vi "Centauro Service Mode Display Checker.vi"(6 "Loop Rate (ms)":u32=250, 7 "Timeout (s)":dbl=5.0 format="%#_13g", 8 "Error In":errorcluster, 9 "Erd_UiLedBitmap ERD #":T1={"ERD Number"=61729, "Data Type"=enum."string"} {"ERD Number" format="%.0x"}, 10 "UI GEA Inputs":T5={"Source"=228, "Destination"=37} {"Destination" format="%.0x"; "Source" format="%.0x"}, 11 "GEA2 Reference In":refnum<k24>) -> (0 "Error Out":errorcluster, 1 "Report Text":string, 2 "LED Status Out":T4, 3 "GEA2 Reference Out":refnum<k24>)   [LabVIEW 2016]
uses:
  Common/LabVIEW GEA2 Toolkit/LabVIEW_GEA2_Toolkit.lvlibp/type defs/Source_Destination.ctl
  Q:/Common/DLLs/GEA3/GeaCommunication.dll
  Common/DLLs/GEA3/GeaCommunication.dll
  Centauro Washer/Product Testcode/Centauro/Valew Common/type defs/LED Status OOB.ctl
  Common/LabVIEW GEA2 Toolkit/LabVIEW_GEA2_Toolkit.lvlibp/type defs/ERD Read Data In.ctl
  Common/LabVIEW GEA2 Toolkit/LabVIEW_GEA2_Toolkit.lvlibp/type defs/Data Type.ctl
  Common/LabVIEW GEA2 Toolkit/LabVIEW_GEA2_Toolkit.lvlibp
panel:
  in  "Board Index":i32
  in  "LED Status Cluster":T4
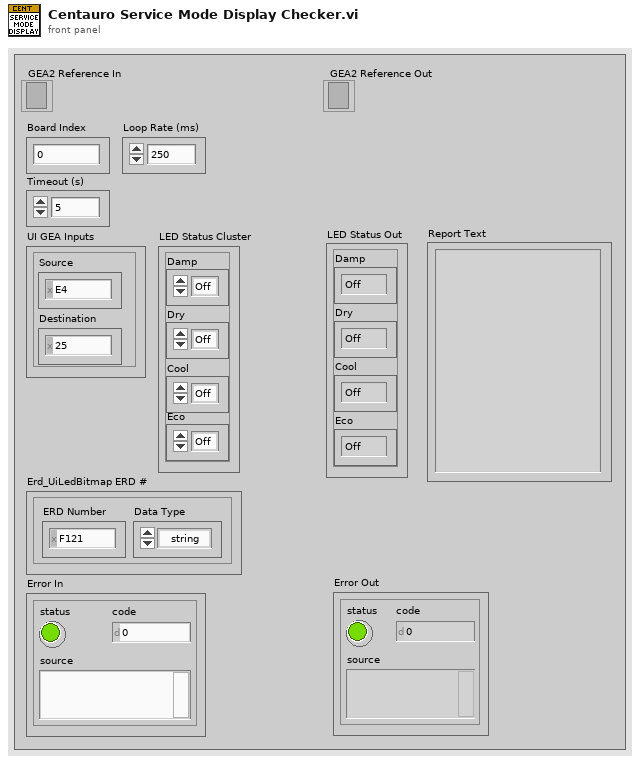
[diagram p1: front panel]
types:
  T1 = typedef "LabVIEW_GEA2_Toolkit.lvlibp/ERD Read Data In.ctl" = cluster{"ERD Number":u16, "Data Type":T2}
  T2 = typedef "LabVIEW_GEA2_Toolkit.lvlibp/Data Type.ctl" = enum16{"string", "boolean", "uint8_t", "uint16_t", "uint32_t", "uint64_t", "int8_t", "int16_t", "int32_t", "int64_t"}
  T3 = typedef "LED Status OOB.ctl" = enum32{"Off", "On", "Blink"}
  T4 = cluster{"Damp":T3, "Dry":T3, "Cool":T3, "Eco":T3}
  T5 = typedef "LabVIEW_GEA2_Toolkit.lvlibp/Source_Destination.ctl" = cluster{"Source":u8, "Destination":u8}
  T6 = enum16{"EQ (==)", "NE (!=)", "GT (>)", "LT (<)", "GE (>=)", "LE (<=)", "GTLT(> <)", "GELE (>= <=)", "GELT (>= <)", "GTLE (> <=)", "LTGT (< >)", "LEGE (<= >=)", "LEGT (<= >)", "LTGE (< >=)", "No Comparison"}
  T7 = typedef "LabVIEW_GEA2_Toolkit.lvlibp/ERD Read Data Out.ctl" = cluster{"ERD Number":u16, "Data":string}
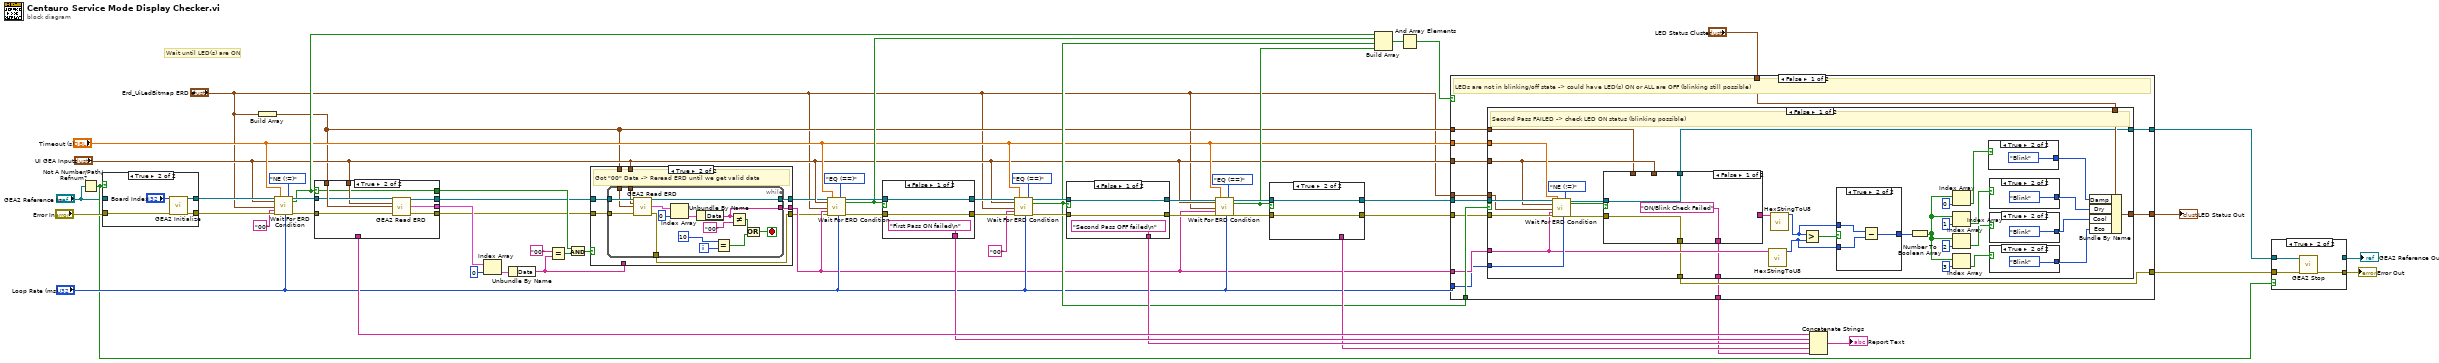
[diagram p0: block diagram]
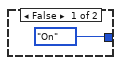
[diagram p4: hidden frame]
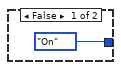
[diagram p5: hidden frame]
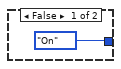
[diagram p6: hidden frame]
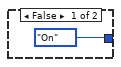
[diagram p7: hidden frame]
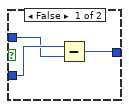
[diagram p8: hidden frame]
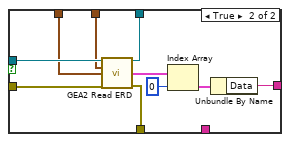
[diagram p9: hidden frame]
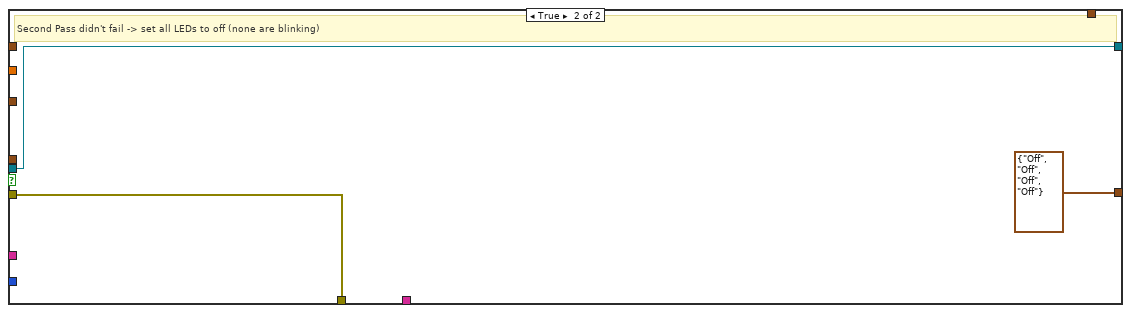
[diagram p10: hidden frame]
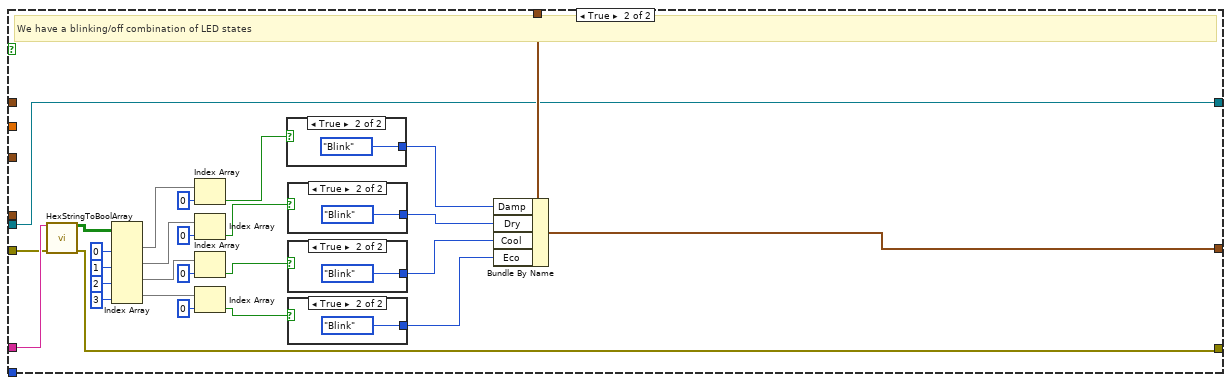
[diagram p11: hidden frame]
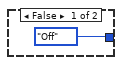
[diagram p12: hidden frame]
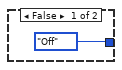
[diagram p13: hidden frame]
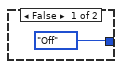
[diagram p14: hidden frame]
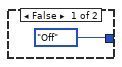
[diagram p15: hidden frame]
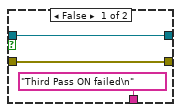
[diagram p16: hidden frame]
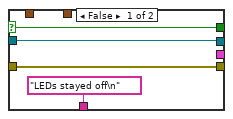
[diagram p20: hidden frame]
diagram:
  # "Wait until LED(s) are ON"
  n1 = Not A Number/Path/Refnum?(number/path/refnum="GEA2 Reference In") -> (NaN/Path/Refnum?=w2:bool)
  n2 = case shown="True" w2 {
    tunnel: [w62 w67] -> w53
    tunnel: "Error In" -> [w62 w66]
    tunnel: [w63 w65] -> w54
    tunnel: "GEA2 Reference In" -> [w63 _]
    frame False {
    }
    frame True {
      n3 = call "GEA2 Initialize.vi"("Board Index"="Board Index", "error in"=w66) -> ("GEA2 Reference Out"=w65:refnum<k24>, "error out"=w67:errorcluster)  [unwired: 11 in, 1 out]
    }
  }
  n4 = Build Array("Erd_UiLedBitmap ERD #") -> (w4:T1[])
  n5 = call "Wait For ERD Condition.vi"("GEA2 Reference In"=w54, "GEA Inputs"="UI GEA Inputs", "ERD Read Data"="Erd_UiLedBitmap ERD #", "Expected Low"="00", "Error In"=w53, "Timeout (s)"="Timeout (s)", "Loop Rate (ms)"="Loop Rate (ms)", "Comparison"=T6."NE (!=)") -> ("GEA2 Reference Out"=w58:refnum<k24>, "Pass/Fail?"=w31:bool, "Error Out"=w57:errorcluster)  [unwired: 7 in, 2 out]
  n6 = case shown="True" w31 {
    selector: w31 -> [w68 w72]
    tunnel: w4 -> [_ w79]
    tunnel: [_ w78] -> w61
    tunnel: [w69 w77] -> w10
    tunnel: w58 -> [w71 w76]
    tunnel: w57 -> [w69 w75]
    tunnel: "UI GEA Inputs" -> [_ w74]
    tunnel: [w71 w73] -> w11
    tunnel: ["LEDs stayed off\n" _] -> w30
    tunnel: [w68 w72] -> w13
    frame False {
    }
    frame True {
      n7 = call "GEA2 Read ERD.vi"("GEA2 Reference In"=w76, "GEA Inputs"=w74, "Read ERD List"=w79, "Error In"=w75) -> ("GEA2 Reference Out"=w73:refnum<k24>, "ERD Data Out"=w78:T7[], "Error Out"=w77:errorcluster)  [unwired: 8 in, 1 out]
    }
  }
  n8 = Index Array(array=w61, index=0) -> (element=w59:T7)
  n9 = Unbundle By Name(w59) -> ("Data"=w8:string)
  n10 = Equal?(x="00", y=w8) -> (x = y?=w14:bool)
  n11 = And(x=w13, y=w14) -> (x .and. y?=w12:bool)
  n12 = case shown="True" w12 {
    tunnel: w11 -> [w81 w89]
    tunnel: w10 -> [w80 w88]
    tunnel: "UI GEA Inputs" -> [_ w87]
    tunnel: w4 -> [_ w86]
    tunnel: [w82 w85] -> w7
    tunnel: w8 -> [w82 _]
    tunnel: [w81 w84] -> w6
    tunnel: [w80 w83] -> w5
    frame False {
      # "Normal data collected -> pass through"
    }
    frame True {
      # "Got \"00\" Data -> Reread ERD until we get valid data"
      n13 = while {
        tunnel: w89 -> [w105]
        tunnel: w88 -> [w104]
        tunnel: w87 -> [w103]
        tunnel: w86 -> [w102]
        tunnel: [w92] -> w85
        tunnel: [w91] -> w84
        tunnel: [w90] -> w83
        i -> [w97]
        stop <- w93 stop-if-true
        n14 = call "GEA2 Read ERD.vi"("GEA2 Reference In"=w105, "GEA Inputs"=w103, "Read ERD List"=w102, "Error In"=w104) -> ("GEA2 Reference Out"=w91:refnum<k24>, "ERD Data Out"=w99:T7[], "Error Out"=w90:errorcluster)  [unwired: 8 in, 1 out]
        n15 = Index Array(array=w99, index=0) -> (element=w100:T7)
        n16 = Unbundle By Name(w100) -> ("Data"=w92:string)
        n17 = Equal?(x=10, y=w97) -> (x = y?=w94:bool)
        n18 = Not Equal?(x=w92, y="00") -> (x != y?=w95:bool)
        n19 = Or(x=w95, y=w94) -> (x .or. y?=w93:bool)
      }
    }
  }
  n20 = call "Wait For ERD Condition.vi"("GEA2 Reference In"=w6, "GEA Inputs"="UI GEA Inputs", "ERD Read Data"="Erd_UiLedBitmap ERD #", "Expected Low"=w7, "Error In"=w5, "Timeout (s)"="Timeout (s)", "Loop Rate (ms)"="Loop Rate (ms)", "Comparison"=T6."EQ (==)") -> ("GEA2 Reference Out"=w49:refnum<k24>, "Pass/Fail?"=w37:bool, "Error Out"=w47:errorcluster)  [unwired: 7 in, 2 out]
  n21 = case shown="False" w37 {
    tunnel: w49 -> [w108 w110]
    tunnel: [w108 w110] -> w48
    tunnel: [w107 w109] -> w46
    tunnel: w47 -> [w107 w109]
    tunnel: ["First Pass ON failed\n" _] -> w29
    frame False {
    }
    frame True {
    }
  }
  n22 = call "Wait For ERD Condition.vi"("GEA2 Reference In"=w48, "GEA Inputs"="UI GEA Inputs", "ERD Read Data"="Erd_UiLedBitmap ERD #", "Expected Low"="00", "Error In"=w46, "Timeout (s)"="Timeout (s)", "Loop Rate (ms)"="Loop Rate (ms)", "Comparison"=T6."EQ (==)") -> ("GEA2 Reference Out"=w44:refnum<k24>, "Pass/Fail?"=w20:bool, "Error Out"=w43:errorcluster)  [unwired: 7 in, 2 out]
  n23 = case shown="False" w20 {
    tunnel: w44 -> [w113 w115]
    tunnel: [w113 w115] -> w41
    tunnel: [w112 w114] -> w40
    tunnel: w43 -> [w112 w114]
    tunnel: ["Second Pass OFF failed\n" _] -> w28
    frame False {
    }
    frame True {
    }
  }
  n24 = call "Wait For ERD Condition.vi"("GEA2 Reference In"=w41, "GEA Inputs"="UI GEA Inputs", "ERD Read Data"="Erd_UiLedBitmap ERD #", "Expected Low"=w7, "Error In"=w40, "Timeout (s)"="Timeout (s)", "Loop Rate (ms)"="Loop Rate (ms)", "Comparison"=T6."EQ (==)") -> ("GEA2 Reference Out"=w39:refnum<k24>, "Pass/Fail?"=w36:bool, "Error Out"=w38:errorcluster)  [unwired: 7 in, 2 out]
  n25 = case shown="True" w36 {
    tunnel: w39 -> [w118 w120]
    tunnel: [w118 w120] -> w22
    tunnel: [w117 w119] -> w33
    tunnel: w38 -> [w117 w119]
    tunnel: ["Third Pass ON failed\n" _] -> w27
    frame False {
    }
    frame True {
    }
  }
  n26 = Build Array(w31, w37, w20, w36) -> (w35:bool[])
  n27 = And Array Elements(Boolean array=w35) -> (logical AND=w34:bool)
  n28 = case shown="False" w34 {
    tunnel: w7 -> [w131 w205]
    tunnel: w33 -> [w129 w204]
    tunnel: [w133 w203] -> w32
    tunnel: [w124 w202] -> w23
    tunnel: w22 -> [w130 w200]
    tunnel: [w122 w200] -> w21
    tunnel: w20 -> [w134 _]
    tunnel: "Timeout (s)" -> [w132 _]
    tunnel: "UI GEA Inputs" -> [w128 _]
    tunnel: "Erd_UiLedBitmap ERD #" -> [w127 _]
    tunnel: "Loop Rate (ms)" -> [w126 _]
    tunnel: w4 -> [w125 _]
    tunnel: "LED Status Cluster" -> [w123 w201]
    tunnel: [w121 _] -> w16
    frame False {
      # "LEDs are not in blinking/off state -> could have LED(s) ON or ALL are OFF (blinking still possible)"
      n29 = case shown="False" w134 {
        tunnel: [w137 T4 {"Damp"=enum."Off", "Dry"=enum."Off", "Cool"=enum."Off", "Eco"=enum."Off"} ("LED Status Cluster")] -> w133
        tunnel: w132 -> [w168 _]
        tunnel: w131 -> [w157 _]
        tunnel: w130 -> [w167 w197]
        tunnel: w129 -> [w166 w198]
        tunnel: w128 -> [w160 _]
        tunnel: w127 -> [w165 _]
        tunnel: w126 -> [w164 _]
        tunnel: w125 -> [w159 _]
        tunnel: [w143 w198] -> w124
        tunnel: w123 -> [w142 _]
        tunnel: [w136 w197] -> w122
        tunnel: [w135 _] -> w121
        frame False {
          # "Second Pass FAILED -> check LED ON status (blinking possible)"
          n30 = call "Wait For ERD Condition.vi"("GEA2 Reference In"=w167, "GEA Inputs"=w160, "ERD Read Data"=w165, "Expected Low"=w157, "Error In"=w166, "Timeout (s)"=w168, "Loop Rate (ms)"=w164, "Comparison"=T6."NE (!=)") -> ("GEA2 Reference Out"=w163:refnum<k24>, "Pass/Fail?"=w162:bool, "Error Out"=w161:errorcluster)  [unwired: 7 in, 2 out]
          n31 = case shown="False" w162 {
            tunnel: w163 -> [w185 w196]
            tunnel: w161 -> [w186 w195]
            tunnel: w160 -> [_ w194]
            tunnel: w159 -> [_ w193]
            tunnel: [_ w189] -> w158
            tunnel: [w186 w188] -> w143
            tunnel: [w185 w187] -> w136
            tunnel: ["ON/Blink Check Failed" _] -> w135
            frame False {
            }
            frame True {
              n32 = call "GEA2 Read ERD.vi"("GEA2 Reference In"=w196, "GEA Inputs"=w194, "Read ERD List"=w193, "Error In"=w195) -> ("GEA2 Reference Out"=w187:refnum<k24>, "ERD Data Out"=w190:T7[], "Error Out"=w188:errorcluster)  [unwired: 8 in, 1 out]
              n33 = Index Array(array=w190, index=0) -> (element=w191:T7)
              n34 = Unbundle By Name(w191) -> ("Data"=w189:string)
            }
          }
          n35 = call "HexStringToU8.vi"("Input String"=w157) -> ("Number Out"=w154:u8)  [unwired: 14 in]
          n36 = call "HexStringToU8.vi"("Input String"=w158) -> ("Number Out"=w155:u8)  [unwired: 14 in]
          n37 = Greater?(x=w155, y=w154) -> (0:w156:bool)
          n38 = case shown="True" w156 {
            tunnel: w155 -> [w179 w183]
            tunnel: w154 -> [w180 w182]
            tunnel: [w178 w181] -> w153
            frame False {
              n39 = Subtract(x=w180, y=w179) -> (x-y=w178:u8)
            }
            frame True {
              n40 = Subtract(x=w183, y=w182) -> (x-y=w181:u8)
            }
          }
          n41 = Number To Boolean Array(number=w153) -> (Boolean array=w148:bool[])
          n42 = Index Array(array=w148, index=0) -> (element=w147:bool)
          n43 = Index Array(array=w148, index=1) -> (element=w146:bool)
          n44 = Index Array(array=w148, index=2) -> (element=w145:bool)
          n45 = Index Array(array=w148, index=3) -> (element=w144:bool)
          n46 = case shown="True" w147 {
            tunnel: [LED_Status_OOB."On" ("Damp") LED_Status_OOB."Blink" ("Damp")] -> w141
            frame False {
            }
            frame True {
            }
          }
          n47 = case shown="True" w146 {
            tunnel: [LED_Status_OOB."On" ("Damp") LED_Status_OOB."Blink" ("Damp")] -> w140
            frame False {
            }
            frame True {
            }
          }
          n48 = case shown="True" w145 {
            tunnel: [LED_Status_OOB."On" ("Damp") LED_Status_OOB."Blink" ("Damp")] -> w139
            frame False {
            }
            frame True {
            }
          }
          n49 = case shown="True" w144 {
            tunnel: [LED_Status_OOB."On" ("Damp") LED_Status_OOB."Blink" ("Damp")] -> w138
            frame False {
            }
            frame True {
            }
          }
          n50 = Bundle By Name(cluster=w142, "Damp"=w141, "Dry"=w140, "Cool"=w139, "Eco"=w138) -> (w137:T4)
        }
        frame True {
          # "Second Pass didn't fail -> set all LEDs to off (none are blinking)"
        }
      }
    }
    frame True {
      # "We have a blinking/off combination of LED states"
      n51 = call "HexStringToBoolArray.vi"("Input String"=w205, "Error In"=w204) -> ("Output Array"=w226:bool[][], "Error Out"=w202:errorcluster)  [unwired: 12 in]
      n52 = Index Array(array=w226, index (col) #1=0 ("disabled index (col)"), index (col) #2=1 ("index (col)"), index (col) #3=2 ("index (col)"), index (col) #4=3 ("index (col)")) -> (element #1=w221:bool[], element #2=w218:bool[], element #3=w214:bool[], element #4=w215:bool[])  [unwired: 4 in]
      n53 = Index Array(array=w221, index=0) -> (element=w213:bool)
      n54 = Index Array(array=w218, index=0) -> (element=w212:bool)
      n55 = Index Array(array=w214, index=0) -> (element=w211:bool)
      n56 = Index Array(array=w215, index=0) -> (element=w210:bool)
      n57 = case shown="True" w213 {
        tunnel: [LED_Status_OOB."Off" ("Damp") LED_Status_OOB."Blink" ("Damp")] -> w209
        frame False {
        }
        frame True {
        }
      }
      n58 = case shown="True" w212 {
        tunnel: [LED_Status_OOB."Off" ("Damp") LED_Status_OOB."Blink" ("Damp")] -> w208
        frame False {
        }
        frame True {
        }
      }
      n59 = case shown="True" w211 {
        tunnel: [LED_Status_OOB."Off" ("Damp") LED_Status_OOB."Blink" ("Damp")] -> w207
        frame False {
        }
        frame True {
        }
      }
      n60 = case shown="True" w210 {
        tunnel: [LED_Status_OOB."Off" ("Damp") LED_Status_OOB."Blink" ("Damp")] -> w206
        frame False {
        }
        frame True {
        }
      }
      n61 = Bundle By Name(cluster=w201, "Damp"=w209, "Dry"=w208, "Cool"=w207, "Eco"=w206) -> (w203:T4)
    }
  }
  "LED Status Out" <- w32
  n62 = Concatenate Strings(w30, w29, w28, w27, w16) -> (→"Report Text":string)
  n63 = case shown="True" w2 {
    tunnel: [w235 w239] -> w25
    tunnel: [w236 _] -> w24
    tunnel: w21 -> [w236 w238]
    tunnel: w23 -> [w235 w237]
    frame False {
    }
    frame True {
      n64 = call "GEA2 Stop.vi"("GEA2 Reference In"=w238, "Error In"=w237) -> ("Error Out"=w239:errorcluster)  [unwired: 13 in]
    }
  }
  "GEA2 Reference Out" <- w24
  "Error Out" <- w25
